vi "Select Point File _ Excel File Merge Same ID Cells.vi"(7 "from template?":bool, 8 "error in":errorcluster caption="错误输入（无错误）", 9 "RowCount":i32, 10 "RowIdx":i32, 11 "report":refnum<class "NI_report.lvclass">) -> (0 "error out":errorcluster caption="错误输出", 3 "report out":refnum<class "NI_report.lvclass">)   [LabVIEW 2016]
uses:
  <vilib>/Utility/NIReport.llb/NI_report.lvclass
  <vilib>/addons/_office/NI_ReportGenerationToolkit.lvlib
  <vilib>/Utility/NIReport.llb/Excel/NI_Excel.lvclass
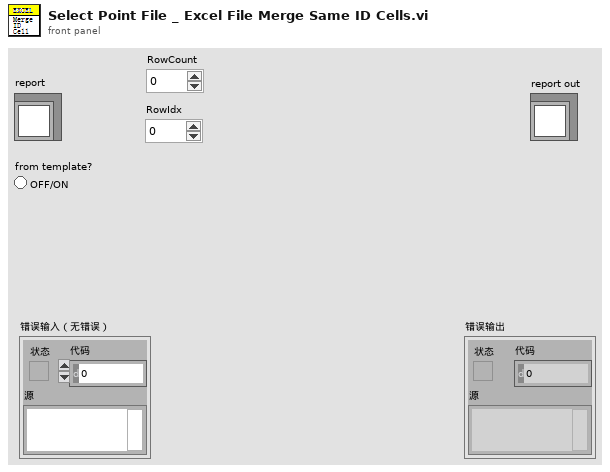
[diagram p1: front panel]
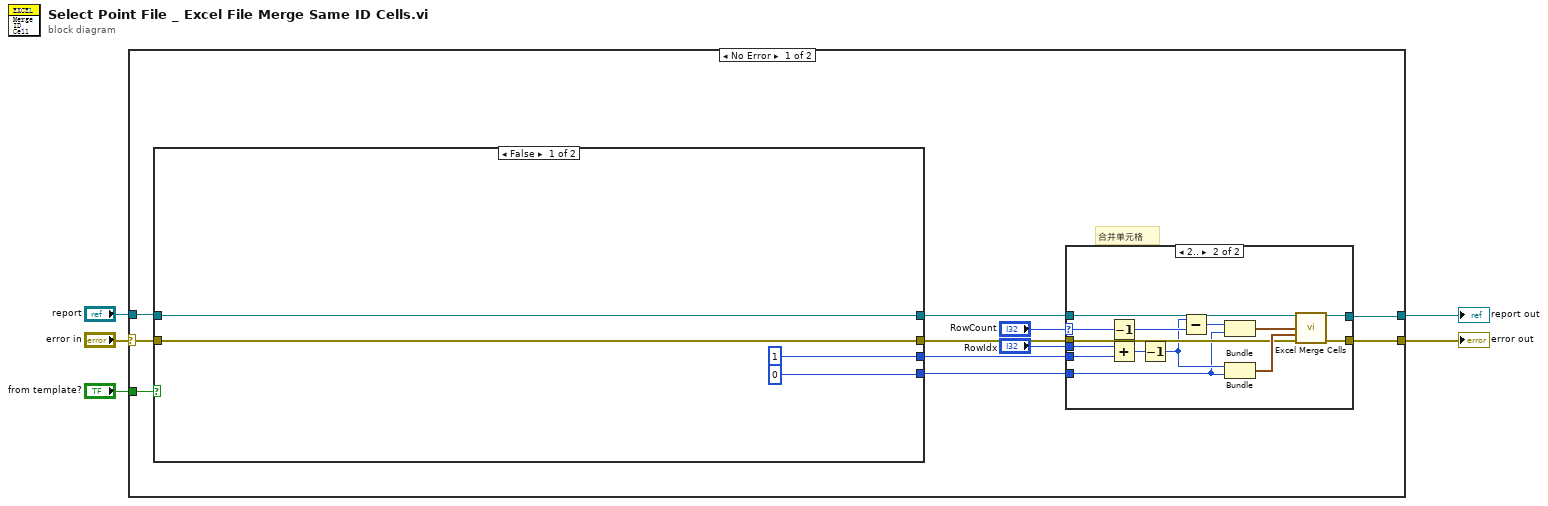
[diagram p0: block diagram]
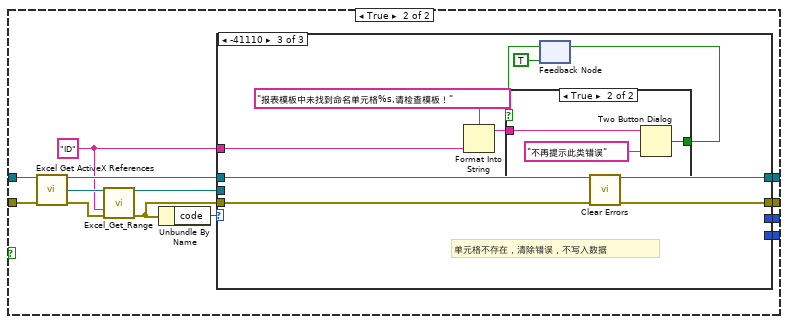
[diagram p3: hidden frame]
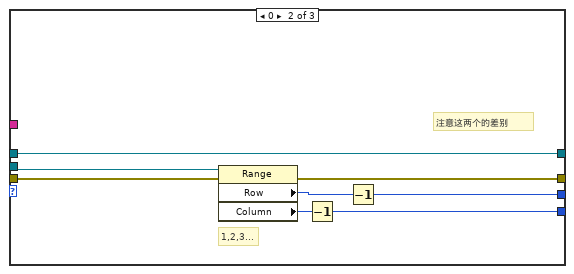
[diagram p5: hidden frame]
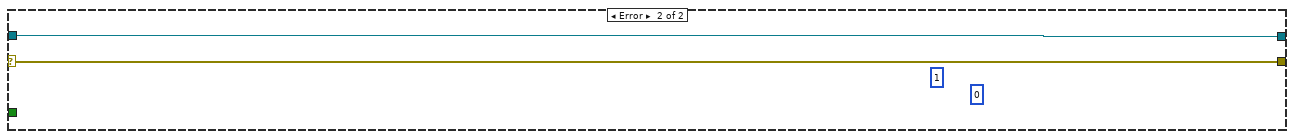
[diagram p7: hidden frame]
diagram:
  n1 = case shown="No Error" "error in" {
    selector: "error in" -> [w16 w74]
    tunnel: [w7 w74] -> w4
    tunnel: "report" -> [w15 w73]
    tunnel: [w8 w73] -> w2
    tunnel: "from template?" -> [w9 _]
    frame No Error {
      # "合并单元格"
      n2 = case shown="False" w9 {
        tunnel: w16 -> [w36 w47]
        tunnel: w15 -> [w33 w48]
        tunnel: [w36 w44] -> w13
        tunnel: [0 w40] -> w10
        tunnel: [1 w39] -> w11
        tunnel: [w33 w37] -> w14
        frame False {
        }
        frame True {
          w38 = "ID"
          n3 = call <vilib>:"Excel Get ActiveX References.vi"("report in"=w48, "error in (no error)"=w47) -> ("report out"=w45:refnum<class "NI_report.lvclass">, "Excel._Worksheet"=w49:refnum<k7>, "error out"=w46:errorcluster)  [unwired: 7 in, 4 out]
          n4 = call <vilib>:"Excel_Get_Range.vi"("Excel._Worksheet"=w49, "name"=w38, "error in (no error)"=w46) -> ("Range"=w42:refnum<k7>, "error out"=w43:errorcluster)  [unwired: 2 in, 9 out]
          n5 = Unbundle By Name(w43) -> ("code"=w41:i32)
          n6 = case shown="-41110" w41 {
            tunnel: w42 -> [_ w59 _]
            tunnel: w43 -> [w50 w58 w67]
            tunnel: w45 -> [w51 w55 w68]
            tunnel: [w51 w55 w68] -> w37
            tunnel: [w50 w54 w66] -> w44
            tunnel: [_ w53 _] -> w40
            tunnel: [_ w52 _] -> w39
            tunnel: w38 -> [_ _ w60]
            frame 1, Default {
            }
            frame 0 {
              # "注意这两个的差别"
              # "1,2,3..."
              n7 = property class="Range"(reference=w59, error in=w58) -> (error out=w54:errorcluster, "Row"=w56:i32, "Column"=w57:i32)  [unwired: 1 out]
              n8 = Decrement(x=w57) -> (x-1=w53:i32)
              n9 = Decrement(x=w56) -> (x-1=w52:i32)
            }
            frame -41110 {
              # "单元格不存在，清除错误，不写入数据"
              n10 = Format Into String(format string="报表模板中未找到命名单元格%s,请检查模板！" ("格式字符串"), w60) -> (resulting string=w65:string)  [unwired: 2 in, 1 out]
              n11 = feedback #1(TRUE) -> (w61:bool)
              n12 = case shown="True" w61 {
                selector: w61 -> [w69 _]
                tunnel: w65 -> [_ w71]
                tunnel: [w69 w70] -> w62
                frame False {
                }
                frame True {
                  n13 = Two Button Dialog(message=w71, 1:"不再提示此类错误" ("F按钮名称（“取消”）")) -> (T button?=w70:bool)  [unwired: 1 in]
                }
              }
              n14 = feedback-in #1(w62) -> ()
              n15 = call <vilib>:"Clear Errors.vi"("error in (no error)"=w67) -> ("error out"=w66:errorcluster)  [unwired: 5 in, 1 out]
            }
          }
        }
      }
      n16 = case shown="2.." "RowCount" {
        selector: "RowCount" -> [_ w27]
        tunnel: w13 -> [w18 w29]
        tunnel: [w18 w28] -> w7
        tunnel: [w17 w19] -> w8
        tunnel: w10 -> [_ w24]
        tunnel: w11 -> [_ w23]
        tunnel: w14 -> [w17 w21]
        tunnel: "RowIdx" -> [_ w20]
        frame 0, 1, Default {
          # "只有一行时不需要进行合并"
        }
        frame 2.. {
          n17 = Decrement(x=w27) -> (x-1=w26:i32)
          n18 = Add(x=w20, y=w23) -> (x+y=w22:i32)
          n19 = Decrement(x=w22) -> (x-1=w25:i32)
          n20 = Subtract(x=w25, y=w26) -> (x-y=w30:i32)
          n21 = Bundle(w30, w24) -> (w31:cluster{i32, i32})  [unwired: 1 in]
          n22 = Bundle(w25, w24) -> (w32:cluster{i32, i32})  [unwired: 1 in]
          n23 = call <vilib>:"Excel Merge Cells.vi"("report in"=w21, "start (-1, -1)"=w31, "end (-1, -1)"=w32, "error in (no error)"=w29) -> ("report out"=w19:refnum<class "NI_report.lvclass">, "error out"=w28:errorcluster)  [unwired: 10 in]
        }
      }
    }
    frame Error {
      (unwired) 1
      (unwired) 0
    }
  }
  "error out" <- w4
  "report out" <- w2
